vi "RIO_ViconReceiver.vi"() -> ()   [LabVIEW 2015]
panel:
  in  "Tab Control":enum32{"Page 1"}(tab)
  out "Rotation":dbl[][](graph)
  out "Translation":dbl[][](graph)
  in  "Stop":bool
  out "x":dbl
  out "z":dbl
  out "y":dbl
  out "roll":dbl
  out "pitch":dbl
  out "yaw":dbl
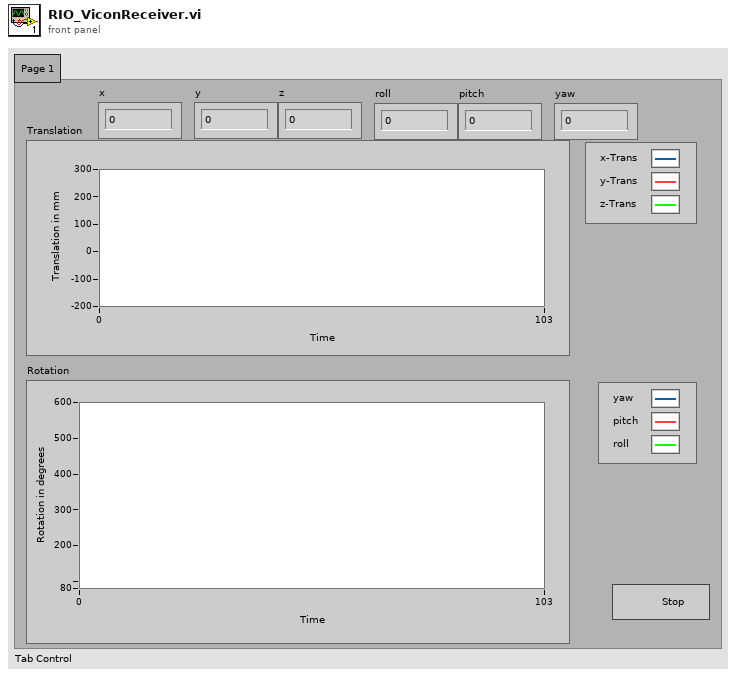
[diagram p1: front panel]
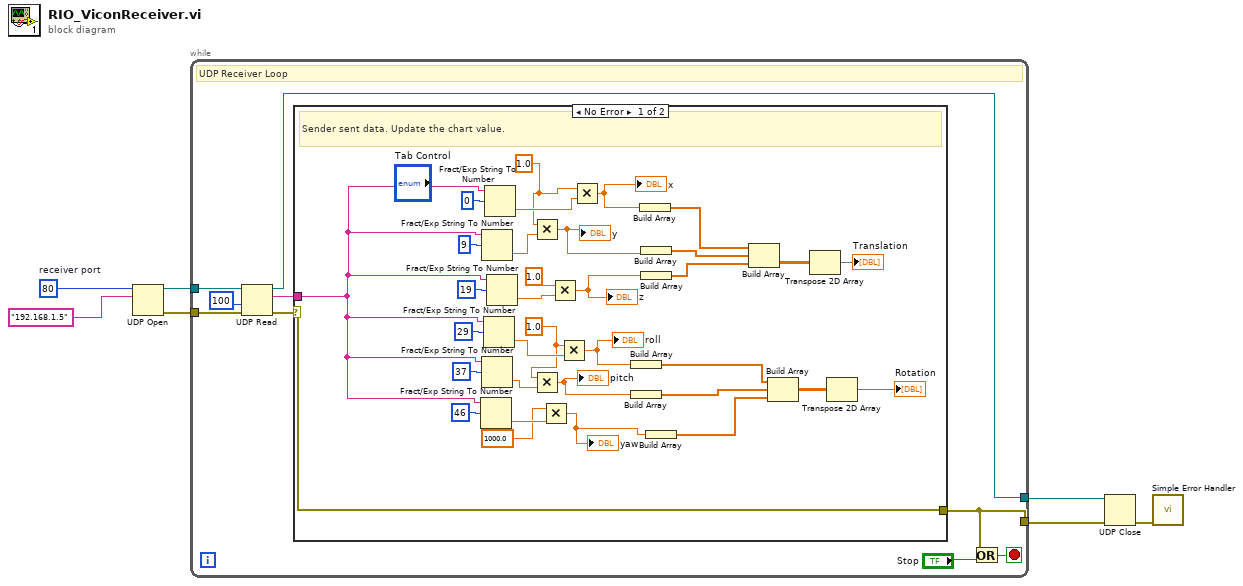
[diagram p0: block diagram]
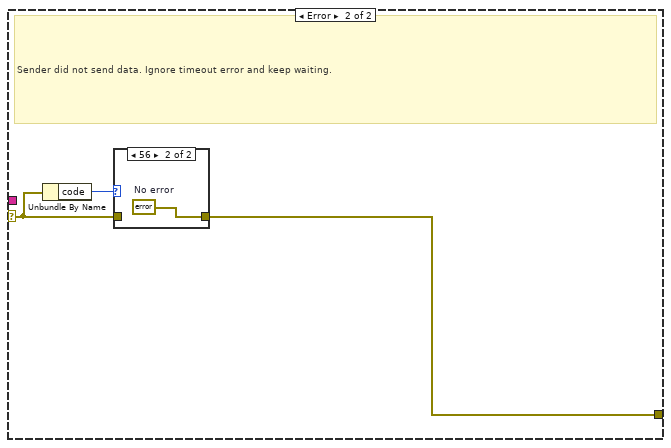
[diagram p2: hidden frame]
diagram:
  w2 = u16 80  # receiver port
  n1 = UDP Open(10:"192.168.1.5" ("service name"), 11:w2) -> (port=w3:refnum<k16>, 0:w4:errorcluster)  [unwired: 3 in, 1 out]
  n2 = while {
    tunnel: w3 -> [w16]
    tunnel: [w8] -> w7
    tunnel: w4 -> [w13]
    tunnel: [w9] -> w5
    stop <- w14 stop-if-true
    # "UDP Receiver Loop"
    n3 = UDP Read(connection ID=w16, timeout ms (25000)=100, 8:w13) -> (data out=w11:string, error out=w10:errorcluster, 3:w8:refnum<k16>)  [unwired: 3 out]
    n4 = case shown="No Error" w10 {
      selector: w10 -> [w50 w52]
      tunnel: w11 -> [w18 _]
      tunnel: [w50 w51] -> w9
      frame No Error {
        w24 = 1.0 ("x")
        w17 = 1.0 ("y")
        # "Sender sent data. Update the chart value."
        n5 = Fract/Exp String To Number(string=w18, offset=46) -> (number=w21:dbl)  [unwired: 2 in, 1 out]
        n6 = Fract/Exp String To Number(string=w18, offset=9) -> (number=w29:dbl)  [unwired: 2 in, 1 out]
        n7 = Fract/Exp String To Number(string=w18, offset=37) -> (number=w23:dbl)  [unwired: 2 in, 1 out]
        n8 = Fract/Exp String To Number(string=w18, offset=29) -> (number=w26:dbl)  [unwired: 2 in, 1 out]
        n9 = Fract/Exp String To Number(string=w18, offset=0) -> (number=w32:dbl)  [unwired: 2 in, 1 out]
        n10 = Fract/Exp String To Number(string=w18, offset=19) -> (number=w31:dbl)  [unwired: 2 in, 1 out]
        n11 = Multiply(x=w17, y=w29) -> (x*y=w28:dbl)
        "y" <- w28
        n12 = Multiply(x=w24, y=w23) -> (x*y=w22:dbl)
        "pitch" <- w22
        n13 = Multiply(x=1000.0, y=w21) -> (x*y=w19:dbl)
        "yaw" <- w19
        n14 = Multiply(x=1.0, y=w31) -> (x*y=w27:dbl)
        "z" <- w27
        n15 = Multiply(x=w24, y=w26) -> (x*y=w25:dbl)
        "roll" <- w25
        n16 = Multiply(x=w17, y=w32) -> (x*y=w33:dbl)
        "x" <- w33
        n17 = Build Array(w25) -> (w36:dbl[])
        n18 = Build Array(w22) -> (w37:dbl[])
        n19 = Build Array(w33) -> (w40:dbl[])
        n20 = Build Array(w28) -> (w39:dbl[])
        n21 = Build Array(w27) -> (w44:dbl[])
        n22 = Build Array(w19) -> (w38:dbl[])
        n23 = Build Array(w40, w39, w44) -> (w46:dbl[][])
        n24 = Build Array(w36, w37, w38) -> (w35:dbl[][])
        n25 = Transpose 2D Array(2D array=w46) -> (transposed array=→"Translation":dbl[][])
        n26 = Transpose 2D Array(2D array=w35) -> (transposed array=→"Rotation":dbl[][])
      }
      frame Error {
        # "Sender did not send data. Ignore timeout error and keep waiting."
        n27 = Unbundle By Name(w52) -> ("code"=w53:i32)
        n28 = case shown="56" w53 {
          tunnel: w52 -> [w54 _]
          tunnel: [w54 w55] -> w51
          frame Default {
          }
          frame 56 {
            w55 = errorcluster {"status"=FALSE, "code"=0, "source"=""}  # No error
          }
        }
      }
    }
    n29 = Or(x=w9, y="Stop") -> (x .or. y?=w14:bool)
  }
  n30 = UDP Close(connection ID=w7, 8:w5) -> (error out=w6:errorcluster)  [unwired: 1 out]
  n31 = call <vilib>:"Simple Error Handler.vi"("error in (no error)"=w6) -> ()  [unwired: 1 in, 8 out]
